vi "Logistic PDF.vi"(9 "b":dbl=1.0, 10 "a":dbl=1.0, 11 "x":dbl) -> (0 "error":i32, 3 "pdf(x)":dbl=0.19661193324148185)   [LabVIEW 2014, in "NI_Gmath.lvlib"]
doc: "Computes the continuous probability density function (PDF) of various distributions. You must manually select the polymorphic instance to use."
uses:
  NI_Gmath.lvlib
  st_error_code.ctl
panel:
  # "Logistic PDF"
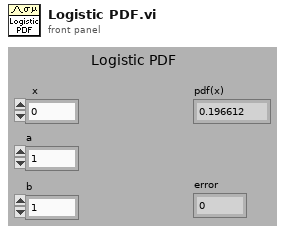
[diagram p1: front panel]
types:
  T1 = typedef "NI_Gmath.lvlib/st_error_code.ctl" = i32
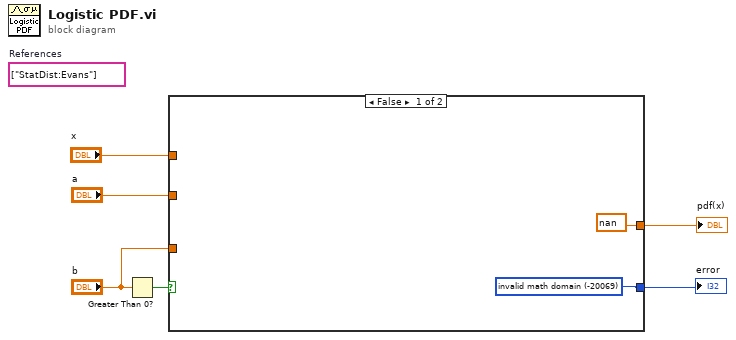
[diagram p0: block diagram]
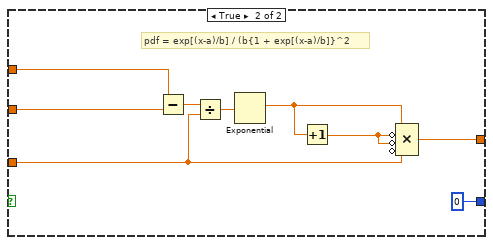
[diagram p2: hidden frame]
diagram:
  (unwired) string[] ["StatDist:Evans"]  # References
  n1 = Greater Than 0?(x="b") -> (x > 0?=w2:bool)
  n2 = case shown="False" w2 {
    tunnel: "b" -> [_ w11]
    tunnel: [w7 0 ("invalid math domain")] -> w6
    tunnel: [nan w14] -> w5
    tunnel: "x" -> [_ w16]
    tunnel: "a" -> [_ w15]
    frame False {
      w7 = T1 -20069 items=["invalid math domain"=-20069, "Fourier interpolation size m >= n"=-20070, "empty array"=-20003] ("stat interp error code")
    }
    frame True {
      # "pdf = exp[(x-a)/b] / (b{1 + exp[(x-a)/b]}^2"
      n3 = Subtract(x=w16, y=w15) -> (x-y=w13:dbl)
      n4 = Divide(x=w13, y=w11) -> (x/y=w12:dbl)
      n5 = Exponential(1:w12) -> (0:w10:dbl)
      n6 = Increment(x=w10) -> (x+1=w9:dbl)
      n7 = Compound Arithmetic op=MULTIPLY(w10, invert w9, invert w9, invert w11) -> (w14:dbl)
    }
  }
  "pdf(x)" <- w5
  "error" <- w6
